vi "FactorialGenerator.vi"(11 "Numeric":u64) -> (3 "Numeric 2":u64)   [LabVIEW 2020]
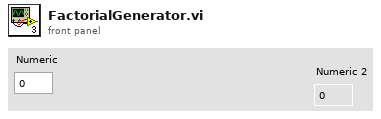
[diagram p1: front panel]
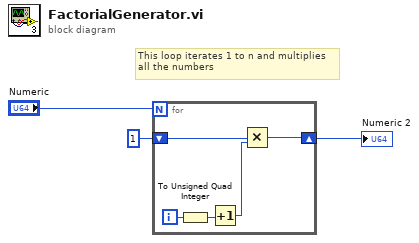
[diagram p0: block diagram]
diagram:
  # "This loop iterates 1 to n and multiplies\nall the numbers"
  n1 = for {
    N: "Numeric" -> [_]
    shift-right: [w7] -> w1
    shift-left: 1 -> [w8]
    i -> [w6]
    n2 = To Unsigned Quad Integer(1:w6) -> (0:w5:u64)
    n3 = Increment(x=w5) -> (x+1=w4:u64)
    n4 = Multiply(x=w8, y=w4) -> (x*y=w7:u64)
  }
  "Numeric 2" <- w1
